vi "ReturnAvailableObjects.vi"(8 "error in (no error)":errorcluster) -> (0 "error out":errorcluster, 3 "Output Array":string[](array[string]))   [LabVIEW 2022 SP3, in "Object_Editor.lvlib" / "Object_Editor.lvclass"]
uses:
  Object_Editor.lvclass
  <userlib>/_OpenG.lib/array/array.llb/Remove Duplicates from 1D Array (String)__ogtk.vi
  Components/ViPER.lvlibp/ViPER.lvclass
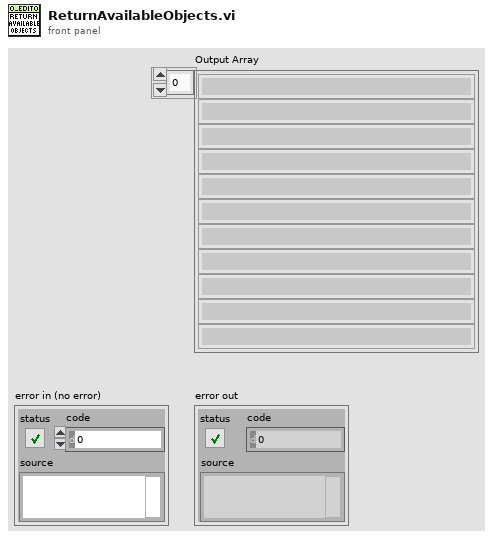
[diagram p1: front panel]
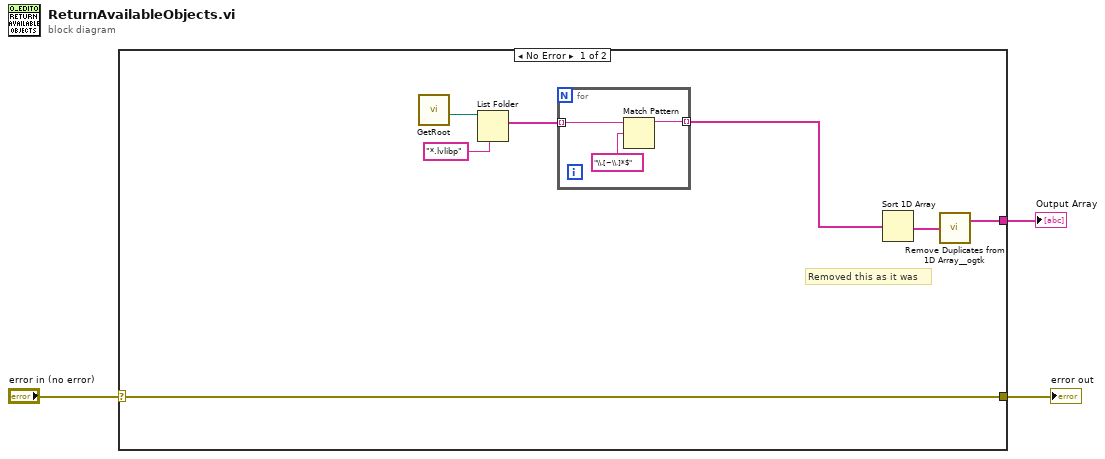
[diagram p0: block diagram]
diagram:
  n1 = case shown="No Error" "error in (no error)" {
    selector: "error in (no error)" -> [w4 w14]
    tunnel: [w7 _] -> w3
    tunnel: [w4 w14] -> w1
    frame No Error {
      # "Removed this as it was"
      n2 = call "GetRoot.vi"() -> ("Root"=w6:path)  [unwired: 10 in, 1 out]
      n3 = List Folder(path=w6, pattern="*.lvlibp") -> (filenames=w9:string[])  [unwired: 2 in, 3 out]
      n4 = for {
        tunnel: w9 -> [w12] mode=indexing
        tunnel: [w11] -> w5 mode=indexing
        n5 = Match Pattern(string=w12, regular expression="\\.[~\\.]*$") -> (before substring=w11:string)  [unwired: 4 out]
      }
      n6 = Sort 1D Array(array=w5) -> (sorted array=w8:string[])
      n7 = call-poly <userlib>:"Remove Duplicates from 1D Array__ogtk.vi"("Input Array"=w8) -> ("Output Array"=w7:string[])  [unwired: 1 out]
    }
    frame Error {
    }
  }
  "Output Array" <- w3
  "error out" <- w1
